vi "Robot Movement Command Interpreter - to rubix.vi"(8 "error in (no error)":errorcluster, 11 "Rbt Cmd":string) -> (0 "error out":errorcluster, 2 "Valid  Cmd?":bool, 3 "Rubix Cmd":T1={"Rotate command"=enum."Middle row left", "Facet to act on"=0})   [LabVIEW 2019]
uses:
  facet and command.ctl
  Cube Data Ops.ctl
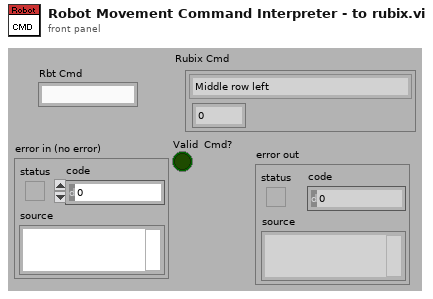
[diagram p1: front panel]
types:
  T1 = typedef "facet and command.ctl" = cluster{"Rotate command":T2, "Facet to act on":u8}
  T2 = typedef "Cube Data Ops.ctl" = enum16{"Initialize", "Set Rubix Ref Array", "Set Rubix Text Array", "Set Current Face", "Get Rubix Text Array", "Generate Rubix Array", "Get Rubix array", "Get Facets to move", "Randomize", "Top row left", "Top row right", "Middle row left", "Middle row right", "Bottom row left", "Bottom row right", "Left column up", "Left column down", "Middle column up", "Middle column down", "Right column up", "Right column down", "Face ccw", "Face cw"}
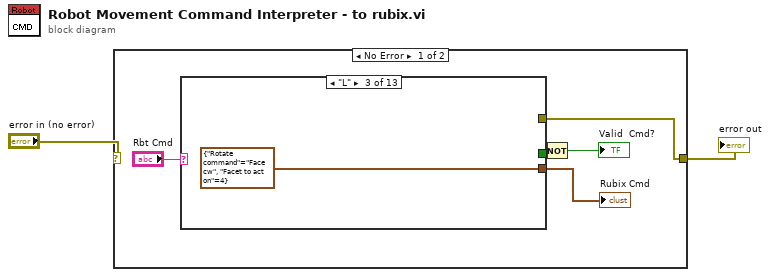
[diagram p0: block diagram]
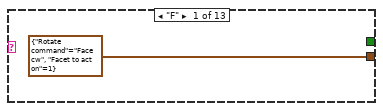
[diagram p2: hidden frame]
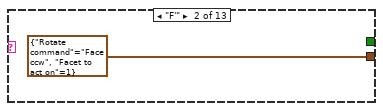
[diagram p3: hidden frame]
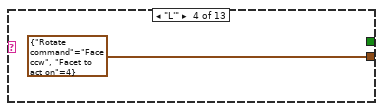
[diagram p4: hidden frame]
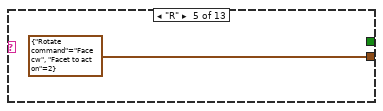
[diagram p5: hidden frame]
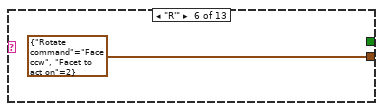
[diagram p6: hidden frame]
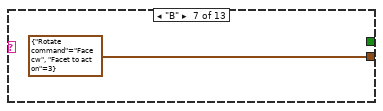
[diagram p7: hidden frame]
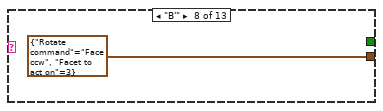
[diagram p8: hidden frame]
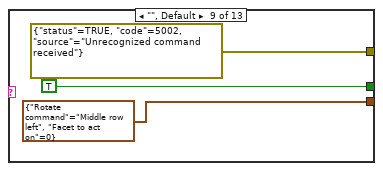
[diagram p9: hidden frame]
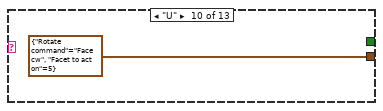
[diagram p10: hidden frame]
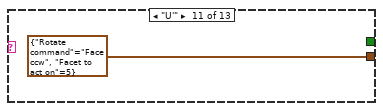
[diagram p11: hidden frame]
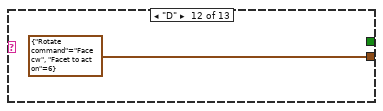
[diagram p12: hidden frame]
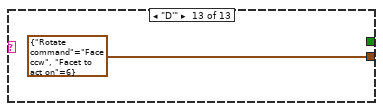
[diagram p13: hidden frame]
diagram:
  n1 = case shown="No Error" "error in (no error)" {
    selector: "error in (no error)" -> [_ w23]
    tunnel: [w4 w23] -> w1
    frame No Error {
      n2 = case shown="\"L\"" "Rbt Cmd" {
        tunnel: [T1 {"Rotate command"=enum."Face cw", "Facet to act on"=1} ("Cluster") T1 {"Rotate command"=enum."Face ccw", "Facet to act on"=1} ("Cluster") T1 {"Rotate command"=enum."Face cw", "Facet to act on"=4} ("Cluster") T1 {"Rotate command"=enum."Face ccw", "Facet to act on"=4} ("Cluster") T1 {"Rotate command"=enum."Face cw", "Facet to act on"=2} ("Cluster") T1 {"Rotate command"=enum."Face ccw", "Facet to act on"=2} ("Cluster") T1 {"Rotate command"=enum."Face cw", "Facet to act on"=3} ("Cluster") T1 {"Rotate command"=enum."Face ccw", "Facet to act on"=3} ("Cluster") T1 {"Rotate command"=enum."Middle row left", "Facet to act on"=0} ("Cluster") T1 {"Rotate command"=enum."Face cw", "Facet to act on"=5} ("Cluster") T1 {"Rotate command"=enum."Face ccw", "Facet to act on"=5} ("Cluster") T1 {"Rotate command"=enum."Face cw", "Facet to act on"=6} ("Cluster") T1 {"Rotate command"=enum."Face ccw", "Facet to act on"=6} ("Cluster")] -> w7
        tunnel: [_ _ _ _ _ _ _ _ TRUE _ _ _ _] -> w6
        tunnel: [_ _ _ _ _ _ _ _ errorcluster {"status"=TRUE, "code"=5002, "source"="Unrecognized command received"} ("error IO") _ _ _ _] -> w4
        frame "F" {
        }
        frame "F'" {
        }
        frame "L" {
        }
        frame "L'" {
        }
        frame "R" {
        }
        frame "R'" {
        }
        frame "B" {
        }
        frame "B'" {
        }
        frame "", Default {
        }
        frame "U" {
        }
        frame "U'" {
        }
        frame "D" {
        }
        frame "D'" {
        }
      }
      "Rubix Cmd" <- w7
      n3 = Not(x=w6) -> (.not. x?=→"Valid  Cmd?":bool)
    }
    frame Error {
    }
  }
  "error out" <- w1
